vi "hc_pair_function.vi"(10 "modelName":string="VVV", 11 "data":dbl[][](array[numeric])) -> (3 "hcPair":dbl[][](array[numeric]))   [LabVIEW 2014]
panel:
  in  "Possible Model Names":string[](array[string])=["E", "V", "EII", "VII", "EEE", "VVV"]
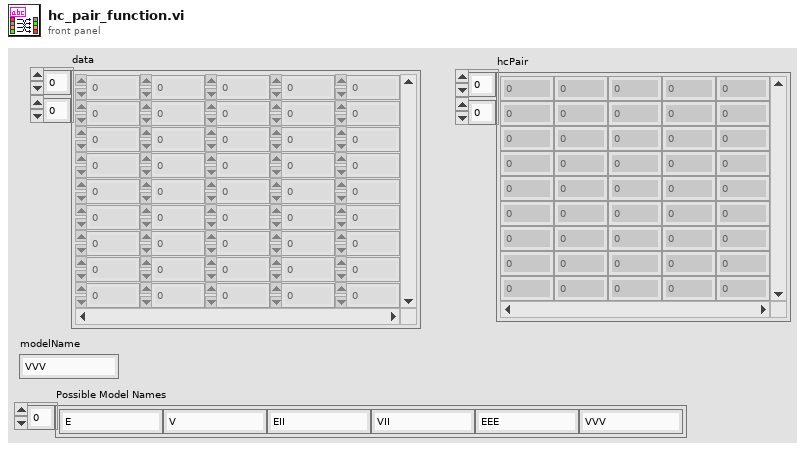
[diagram p1: front panel]
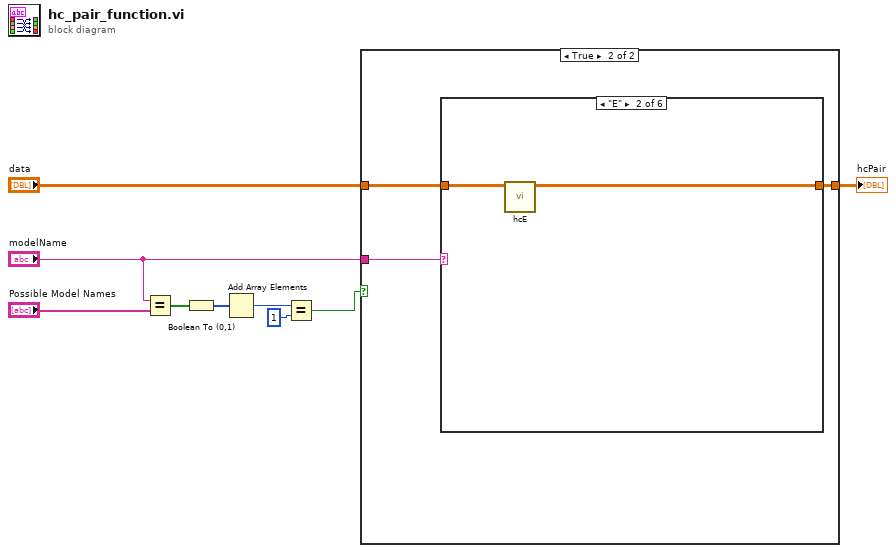
[diagram p0: block diagram]
diagram:
  n1 = Equal?(x="modelName", y="Possible Model Names") -> (x = y?=w5:bool[])
  n2 = Boolean To (0,1)(Boolean=w5) -> (0, 1=w6:i16[])
  n3 = Add Array Elements(numeric array=w6) -> (sum=w7:i16)
  n4 = Equal?(x=w7, y=i16 1) -> (x = y?=w2:bool)
  n5 = case shown="True" w2 {
    tunnel: "modelName" -> [_ w12]
    tunnel: "data" -> [_ w11]
    tunnel: [_ w10] -> w1
    frame False {
    }
    frame True {
      n6 = case shown="\"E\"" w12 {
        tunnel: w11 -> [_ w14 _ _ _ _]
        tunnel: [_ w13 _ _ _ _] -> w10
        frame "VVV", Default {
        }
        frame "E" {
          n7 = call "hcE.vi"("data"=w14) -> ("hcPair"=w13:dbl[][])  [unwired: 7 in, 3 out]
        }
        frame "V" {
        }
        frame "EII" {
        }
        frame "VII" {
        }
        frame "EEE" {
        }
      }
    }
  }
  "hcPair" <- w1
